vi "Close sync interface.vi"(0 "TPDO 4 object in":refnum<k20>, 1 "TPDO 3 object in":refnum<k20>, 2 "TPDO 2 object in":refnum<k20>, 3 "TPDO 1 object in":refnum<k20>, 4 "SYNC object in":refnum<k20>, 5 "error in (no error)":errorcluster) -> (19 "error out":errorcluster)   [LabVIEW 2016]
uses:
  <vilib>/CANopenLib/CANOPEN.llb/CANopen TPDO Close.vi
  <vilib>/CANopenLib/CANOPEN.llb/CANopen SYNC Close.vi
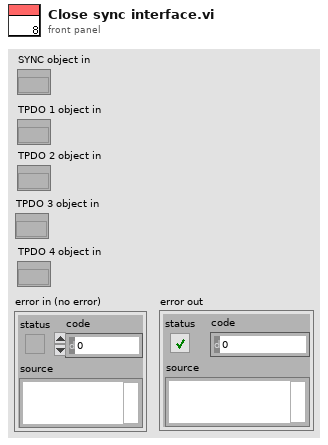
[diagram p1: front panel]
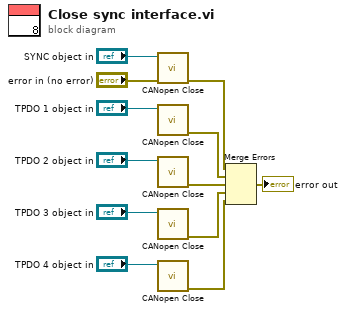
[diagram p0: block diagram]
diagram:
  n1 = call-poly <vilib>:"CANopen Close.vi"("error in (no error)"="error in (no error)", "SYNC object in"="SYNC object in") -> ("error out"=w7:errorcluster)  [unwired: 9 in]
  n2 = call-poly <vilib>:"CANopen Close.vi"("TPDO object in"="TPDO 1 object in") -> ("error out"=w6:errorcluster)  [unwired: 10 in]
  n3 = call-poly <vilib>:"CANopen Close.vi"("TPDO object in"="TPDO 2 object in") -> ("error out"=w5:errorcluster)  [unwired: 10 in]
  n4 = call-poly <vilib>:"CANopen Close.vi"("TPDO object in"="TPDO 3 object in") -> ("error out"=w4:errorcluster)  [unwired: 10 in]
  n5 = call-poly <vilib>:"CANopen Close.vi"("TPDO object in"="TPDO 4 object in") -> ("error out"=w3:errorcluster)  [unwired: 10 in]
  n6 = Merge Errors(w7, w6, w5, w4, w3) -> (→"error out":errorcluster)
